vi "Get XML Encoding.vi"(8 "error in (no error)":errorcluster, 10 "XML string":string) -> (0 "error out":errorcluster, 1 "Encoding":string, 2 "XML string out":string)   [LabVIEW 2013]
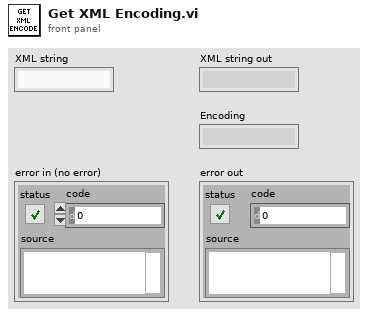
[diagram p1: front panel]
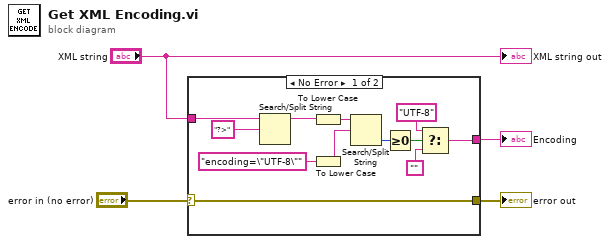
[diagram p0: block diagram]
diagram:
  n1 = case shown="No Error" "error in (no error)" {
    selector: "error in (no error)" -> [w5 w17]
    tunnel: "XML string" -> [w6 _]
    tunnel: [w7 _] -> w2
    tunnel: [w5 w17] -> w4
    frame No Error {
      n2 = Search/Split String(string=w6, search string/char (-)="?>" ("regular expression")) -> (substring before match=w15:string)  [unwired: 1 in, 2 out]
      n3 = To Lower Case(string=w15) -> (all lower case string=w13:string)
      n4 = To Lower Case(string="encoding=\"UTF-8\"") -> (all lower case string=w12:string)
      n5 = Search/Split String(string=w13, search string/char (-)=w12) -> (offset of match=w11:i32)  [unwired: 1 in, 2 out]
      n6 = Greater Or Equal To 0?(x=w11) -> (x >= 0?=w10:bool)
      n7 = Select(t="UTF-8" ("string"), s=w10, f="") -> (s? t:f=w7:string)
    }
    frame Error {
    }
  }
  "error out" <- w4
  "Encoding" <- w2
  "XML string out" <- "XML string"
